vi "Graphics-Draw Angle (Picture).vi"(0 "picture in":picture, 7 "rect":T1, 11 "point left":bool, 12 "color(black)":u32(colorbox)=16711680, 13 "pen":T2) -> (4 "picture out":picture)   [LabVIEW 2020]
uses:
  <vilib>/Utility/miscctls.llb/LVRectTypeDef.ctl
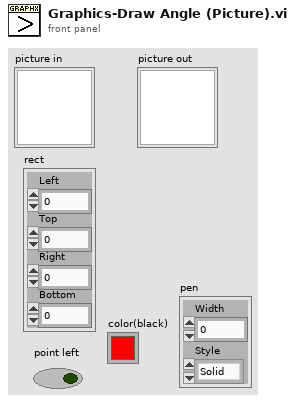
[diagram p1: front panel]
types:
  T1 = typedef "LVRectTypeDef.ctl" = cluster{"Left":i16, "Top":i16, "Right":i16, "Bottom":i16}
  T2 = cluster{"Width":u16, "Style":enum32{"Solid", "Dash", "Dot", "DashDot", "DashDotDot"}}
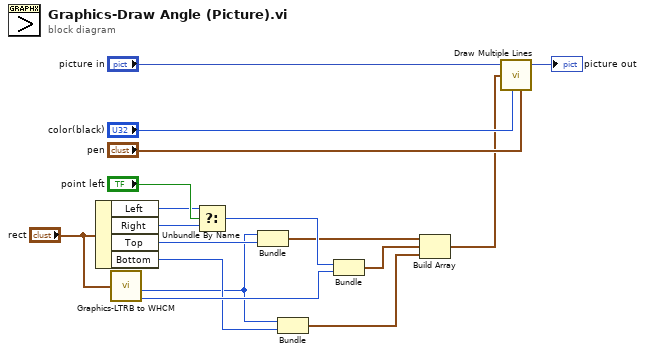
[diagram p0: block diagram]
diagram:
  n1 = Unbundle By Name("rect") -> ("Left"=w10:i16, "Right"=w11:i16, "Top"=w12:i16, "Bottom"=w8:i16)
  n2 = call "Graphics-LTRB to WHCM.vi"("LTRB"="rect") -> ("Middle"=w9:i16, "Center"=w7:i16)  [unwired: 4 in, 2 out]
  n3 = Select(t=w10, s="point left", f=w11) -> (s? t:f=w6:i16)
  n4 = Bundle("Center"=w7, "Top"=w12) -> (w4:cluster{"Center":i16, "Top":i16})  [unwired: 1 in]
  n5 = Bundle("Center"=w7, "Bottom"=w8) -> (w2:cluster{"Center":i16, "Bottom":i16})  [unwired: 1 in]
  n6 = Bundle("Right"=w6, "Middle"=w9) -> (w3:cluster{"Right":i16, "Middle":i16})  [unwired: 1 in]
  n7 = Build Array(w4, w3, w2) -> (w1:cluster{"Center":i16, "Bottom":i16}[])
  n8 = call <vilib>:"Draw Multiple Lines.vi"("picture"="picture in", "line endpoints"=w1, "color(black)"="color(black)", "pen"="pen") -> ("new picture"=→"picture out":picture)  [unwired: 5 in]
